vi "Knock.vi"(8 "error in (no error)":errorcluster, 11 "Node Ptr":T3 format="%.0x") -> (0 "error out":errorcluster)   [LabVIEW 2016, in "DCM System Explorer.lvlib"]
uses:
  DCM System Explorer.lvlib
  <vilib>/NI Veristand/Custom Device API/Custom Device Item Ref.ctl
  Shared/DCM Properties.vi
  Shared/DCM Constants and GUIDs.vi
  <vilib>/NI Veristand/Custom Device Tools/Custom Device Utility Library/NI VeriStand - Search for Item by Name.vi
  <vilib>/NI VeriStand/Custom Device API/Custom Device API.lvlib
  DCM Shared.lvlib
  <vilib>/NI Veristand/Custom Device Tools/Custom Device Utility Library/Custom Device Utility Library.lvlib
panel:
  in  "Settings":T1={"Knock Sensor"=[0, 0, 0, 0, 0, 0, 0, 0, 0, 0, 0, 0, 0, 0, 0, 0], "Knock Offset [CAD]"=[0.0, 0.0, 0.0, 0.0, 0.0, 0.0, 0.0, 0.0, 0.0, 0.0, 0.0, 0.0, 0.0, 0.0, 0.0, 0.0]} {"Knock Sensor" items=["Sensor 1", "Sensor 2", "Sensor 3", "Sensor 4", "Sensor 5", "Sensor 6", "Sensor 7", "Sensor 8", "Sensor 9", "Sensor 10", "Sensor 11", "Sensor 12"]}
  in  "Controls":T2={"Low Cutoff [Hz]"=5000.0, "High Cutoff [Hz]"=6000.0, "Threshold"=2.0, "Knock Start [CAD]"=0.0, "Knock End [CAD]"=0.0, "Reference End [CAD]"=0.0, "Reference Start [CAD]"=0.0} {"High Cutoff [Hz]" format="%#_6p"; "Low Cutoff [Hz]" format="%#_6p"}
  in  "Header":cluster{"Section Name":string}={"Section Name"="Knock Setup"}
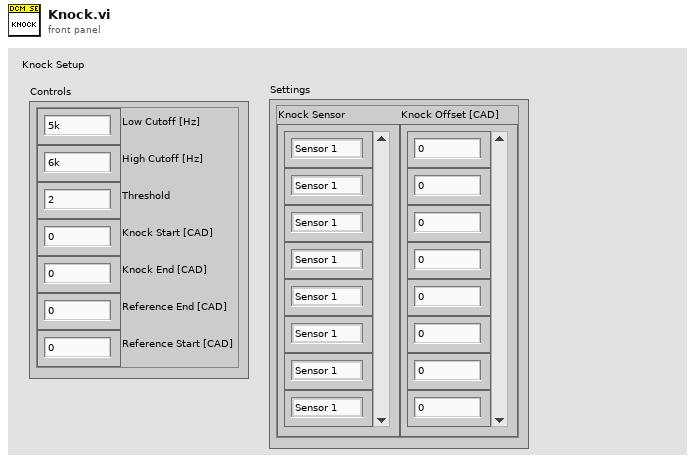
[diagram p1: front panel]
types:
  T1 = cluster{"Knock Sensor":i32[], "Knock Offset [CAD]":sgl[]}
  T2 = cluster{"Low Cutoff [Hz]":sgl, "High Cutoff [Hz]":sgl, "Threshold":sgl, "Knock Start [CAD]":sgl, "Knock End [CAD]":sgl, "Reference End [CAD]":sgl, "Reference Start [CAD]":sgl}
  T3 = typedef "Custom Device API.lvlib/Custom Device Item Ref.ctl" = u64
  T4 = typedef "DCM Shared.lvlib/Channel.ctl" = cluster{"Name":string, "Units":string, "Default":dbl, "Description":string}
  T5 = typedef "Custom Device API.lvlib/Custom Device Channel.ctl" = cluster{"Type":T6, "Units":string, "Default Value":dbl, "Faultable":bool, "Scalable":bool}
  T6 = typedef "Custom Device API.lvlib/Custom Device Channel Type.ctl" = enum16{"Input", "Output"}
  T7 = cluster{"[0]":dbl, "[1]":dbl, "[2]":dbl, "[3]":dbl, "[4]":dbl, "[5]":dbl, "[6]":dbl}
  T8 = typedef "Custom Device API.lvlib/Custom Device Commands.ctl" = enum16{"Default", "Item renamed", "Shutdown", "Dynamic button pressed"}
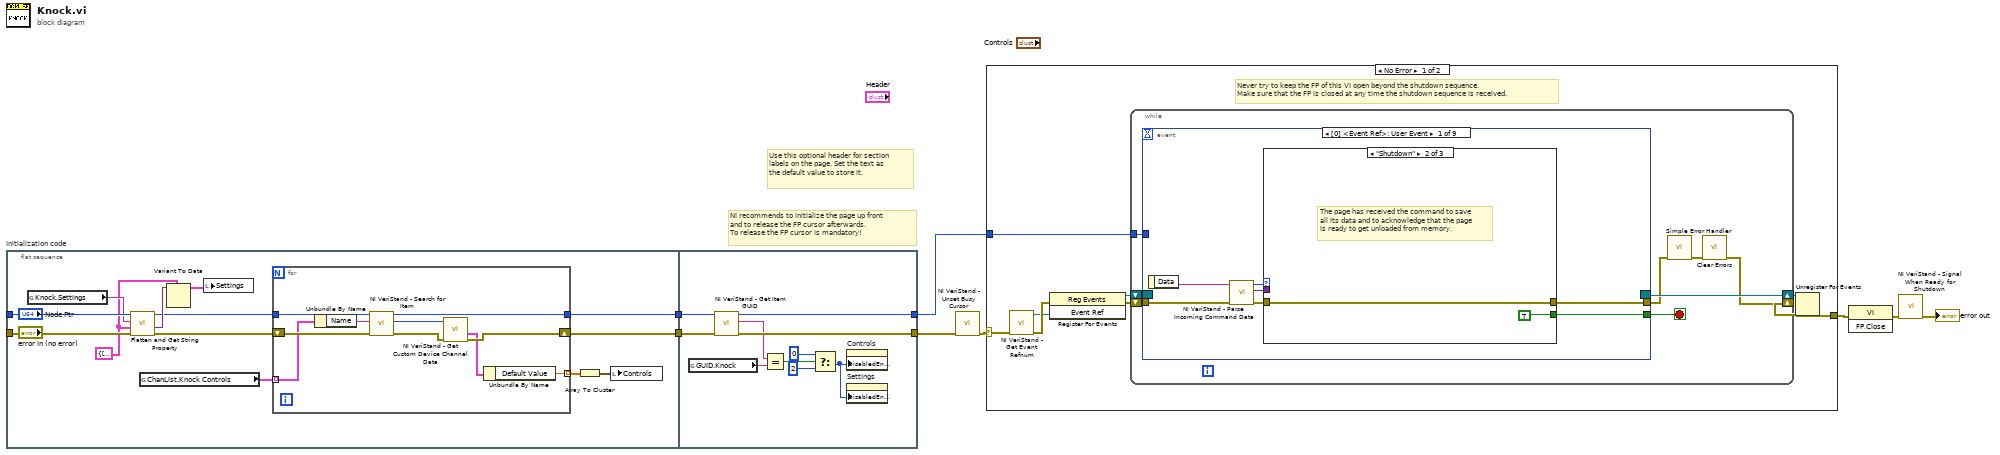
[diagram p0: block diagram]
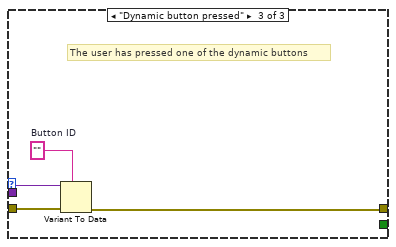
[diagram p3: hidden frame]
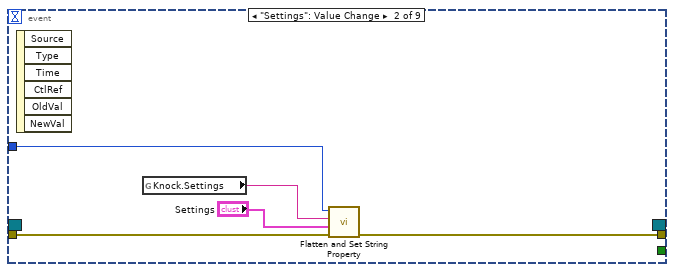
[diagram p4: hidden frame]
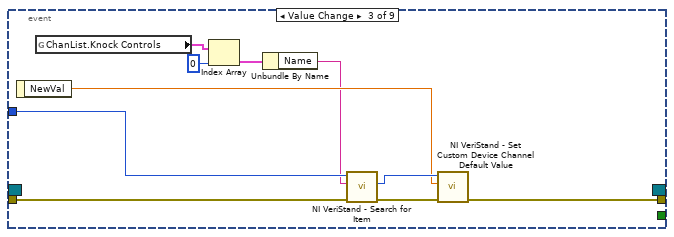
[diagram p5: hidden frame]
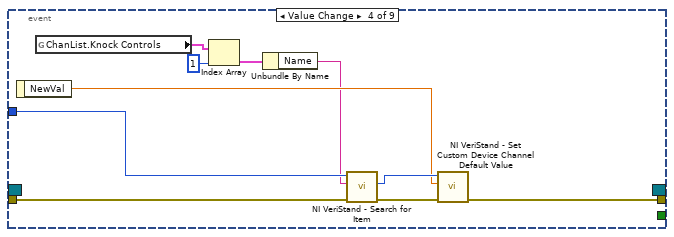
[diagram p6: hidden frame]
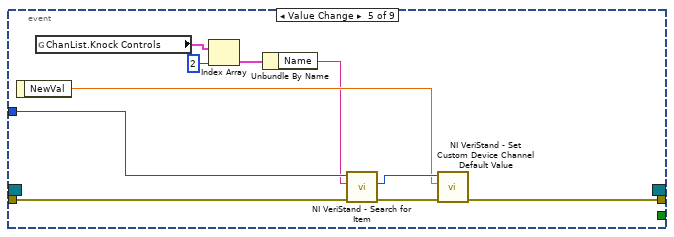
[diagram p7: hidden frame]
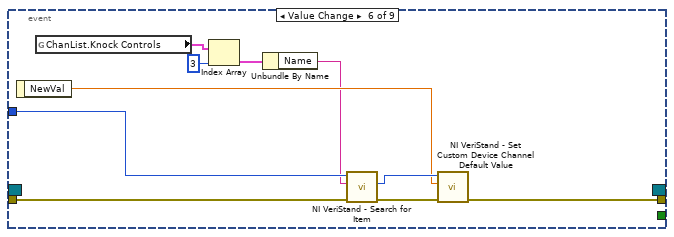
[diagram p8: hidden frame]
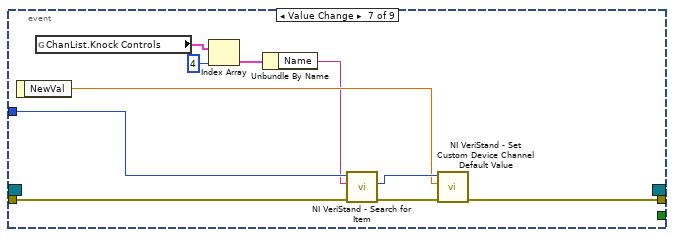
[diagram p9: hidden frame]
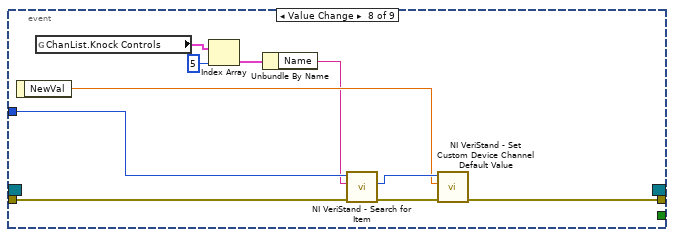
[diagram p10: hidden frame]
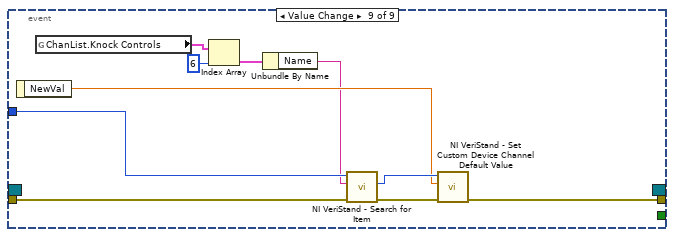
[diagram p11: hidden frame]
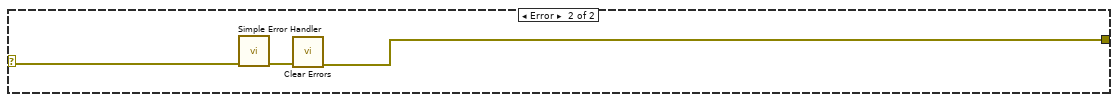
[diagram p12: hidden frame]
diagram:
  # "Use this optional header for section labels on the page. Set the text as the default value to store it."
  # "NI recommends to initialize the page up front\nand to release the FP cursor afterwards.\nTo release the FP cursor is mandatory!"
  n1 = flat-sequence "Initialization code" {
    tunnel: "error in (no error)" -> [w22]
    tunnel: "Node Ptr" -> [w21]
    tunnel: [w18] -> w2
    tunnel: [w17] -> w1
    tunnel: [w40] -> w3
    tunnel: [w41] -> w4
    tunnel: w2 -> [w43]
    tunnel: w1 -> [w42]
    frame #0 {
      w12 = T1 {"Knock Sensor"=[0, 0, 0, 0, 0, 0, 0, 0, 0, 0, 0, 0, 0, 0, 0, 0], "Knock Offset [CAD]"=[0.0, 0.0, 0.0, 0.0, 0.0, 0.0, 0.0, 0.0, 0.0, 0.0, 0.0, 0.0, 0.0, 0.0, 0.0, 0.0]} ("Settings")
      n2 = global read "DCM Properties.vi" "Knock.Settings"() -> (w20:string)
      n3 = call "Flatten and Get String Property.vi"("error in (no error)"=w22, "Default Value"=w12, "Property Name"=w20, "Section Ref in"=w21) -> ("error out"=w16:errorcluster, "Value"=w23:variant, "Section Ref out"=w19:T3)  [unwired: 5 in]
      n4 = global read "DCM Constants and GUIDs.vi" "ChanList.Knock Controls"() -> (w15:T4[])
      n5 = Variant To Data(type=w12, Variant=w23) -> (data=w11:T1)  [unwired: 1 in, 1 out]
      n6 = local write "Settings"(w11) -> ()
      n7 = for {
        tunnel: w19 -> [w33]
        tunnel: [w31] -> w18
        shift-right: [w26] -> w17
        shift-left: w16 -> [w32]
        tunnel: w15 -> [w30] mode=indexing
        tunnel: [w24] -> w14 mode=indexing
        n8 = Unbundle By Name(w30) -> ("Name"=w29:string)
        n9 = call-poly <vilib>:"NI VeriStand - Search for Item.vi"("error in"=w32, "Item Name"=w29, "Section Ref in"=w33) -> ("error out"=w28:errorcluster, "Item Ref"=w27:T3, "Section Ref out"=w31:T3)  [unwired: 5 in, 1 out]
        n10 = call <vilib>:"NI VeriStand - Get Custom Device Channel Data.vi"("error in (no error)"=w28, "Channel Ref in"=w27) -> ("error out"=w26:errorcluster, "Channel"=w25:T5)  [unwired: 4 in, 4 out]
        n11 = Unbundle By Name(w25) -> ("Default Value"=w24:dbl)
      }
      n12 = Array To Cluster(array=w14) -> (cluster=w13:T7)
      n13 = local write "Controls"(w13) -> ()
    }
    frame #1 {
      n14 = global read "DCM Constants and GUIDs.vi" "GUID.Knock"() -> (w39:string)
      n15 = call <vilib>:"NI VeriStand - Get Item GUID.vi"("error in (no error)"=w42, "Item Ref in"=w43) -> ("error out"=w40:errorcluster, "GUID"=w38:string, "Item Ref out"=w41:T3)  [unwired: 7 in]
      n16 = Equal?(x=w38, y=w39) -> (x = y?=w35:bool)
      n17 = Select(t=0, s=w35, f=2) -> (s? t:f=w34:i32)
      n18 = property on="Controls" class="Clust (strict)"("DisabledEnum"=w34) -> ()  [unwired: 2 in, 2 out]
      n19 = property on="Settings" class="Clust (strict)"("DisabledEnum"=w34) -> ()  [unwired: 2 in, 2 out]
    }
  }
  n20 = call <vilib>:"NI VeriStand - Unset Busy Cursor.vi"("error in (no error)"=w3) -> ("error out"=w6:errorcluster)  [unwired: 10 out]
  n21 = case shown="No Error" w6 {
    selector: w6 -> [w45 w152]
    tunnel: [w49 w150] -> w10
    tunnel: w4 -> [w44 _]
    frame No Error {
      # "Never try to keep the FP of this VI open beyond the shutdown sequence.\nMake sure that the FP is closed at any time the shutdown sequence is received."
      n22 = call <vilib>:"NI VeriStand - Get Event Refnum.vi"("error in (no error)"=w45) -> ("error out"=w52:errorcluster, "Event Ref"=w48:refnum<user-event>)  [unwired: 9 out]
      n23 = register-events(error in=w52, w48) -> (reference out=w46:refnum<event-registration>, error out=w47:errorcluster)  [unwired: 1 in]
      n24 = while {
        shift-right: [w54] -> w50
        shift-left: w47 -> [w59]
        shift-right: [w60] -> w51
        shift-left: w46 -> [w58]
        tunnel: w44 -> [w53]
        stop <- w57 stop-if-true
        n25 = event shown="[0] <Event Ref>: User Event" {
          selector: w58 -> [_ _ _ _ _ _ _ _ _]
          dyn-events: [_ _ _ _ _ _ _ _ _] -> w60
          timeout: _ -> [_ _ _ _ _ _ _ _ _]
          tunnel: w59 -> [w67 w79 w87 w97 w107 w117 w127 w137 w147]
          tunnel: [w63 _ _ _ _ _ _ _ _] -> w57
          tunnel: [w62 w78 w89 w99 w109 w119 w129 w139 w149] -> w56
          tunnel: w53 -> [_ w77 w88 w98 w108 w118 w128 w138 w148]
          event User Event {
            n26 = event-data() -> ("Data"=w66:string)  [unwired: 1 out]
            n27 = call <vilib>:"NI VeriStand - Parse Incoming Command Data.vi"("error in (no error)"=w67, "Incoming data"=w66) -> ("error out"=w65:errorcluster, "Outgoing data"=w61:variant, "Action"=w64:T8)  [unwired: 7 out]
            n28 = case shown="\"Shutdown\"" w64 {
              tunnel: w65 -> [w68 w69 w74]
              tunnel: [_ TRUE _] -> w63
              tunnel: [w68 w69 w71] -> w62
              tunnel: w61 -> [_ _ w73]
              frame "Default", Default {
              }
              frame "Shutdown" {
                # "The page has received the command to save all its data and to acknowledge that the page is ready to get unloaded from memory."
              }
              frame "Dynamic button pressed" {
                w72 = ""  # Button ID
                # "The user has pressed one of the dynamic buttons"
                n29 = Variant To Data(error in=w74, type=w72, Variant=w73) -> (error out=w71:errorcluster)  [unwired: 1 out]
              }
            }
          }
          event "Settings": Value Change {
            n30 = event-data() -> ()  [unwired: 7 out]
            n31 = global read "DCM Properties.vi" "Knock.Settings"() -> (w76:string)
            n32 = call "Flatten and Set String Property.vi"("error in (no error)"=w79, "Value"="Settings", "Property Name"=w76, "Section Ref in"=w77) -> ("error out"=w78:errorcluster)  [unwired: 6 in, 1 out]
          }
          event "Controls.Low Cutoff [Hz]": Value Change {
            n33 = event-data() -> ("NewVal"=w84:sgl)  [unwired: 1 out]
            n34 = global read "DCM Constants and GUIDs.vi" "ChanList.Knock Controls"() -> (w83:T4[])
            n35 = Index Array(array=w83, index=0) -> (element=w81:T4)
            n36 = Unbundle By Name(w81) -> ("Name"=w80:string)
            n37 = call-poly <vilib>:"NI VeriStand - Search for Item.vi"("error in"=w87, "Item Name"=w80, "Section Ref in"=w88) -> ("error out"=w86:errorcluster, "Item Ref"=w85:T3)  [unwired: 5 in, 2 out]
            n38 = call <vilib>:"NI VeriStand - Set Custom Device Channel Default Value.vi"("error in (no error)"=w86, "Default Value"=w84, "Channel Ref in"=w85) -> ("error out"=w89:errorcluster)  [unwired: 7 in, 1 out]
          }
          event "Controls.High Cutoff [Hz]": Value Change {
            n39 = event-data() -> ("NewVal"=w94:sgl)  [unwired: 1 out]
            n40 = global read "DCM Constants and GUIDs.vi" "ChanList.Knock Controls"() -> (w93:T4[])
            n41 = Index Array(array=w93, index=1) -> (element=w91:T4)
            n42 = Unbundle By Name(w91) -> ("Name"=w90:string)
            n43 = call-poly <vilib>:"NI VeriStand - Search for Item.vi"("error in"=w97, "Item Name"=w90, "Section Ref in"=w98) -> ("error out"=w96:errorcluster, "Item Ref"=w95:T3)  [unwired: 5 in, 2 out]
            n44 = call <vilib>:"NI VeriStand - Set Custom Device Channel Default Value.vi"("error in (no error)"=w96, "Default Value"=w94, "Channel Ref in"=w95) -> ("error out"=w99:errorcluster)  [unwired: 7 in, 1 out]
          }
          event "Controls.Threshold": Value Change {
            n45 = event-data() -> ("NewVal"=w104:sgl)  [unwired: 1 out]
            n46 = global read "DCM Constants and GUIDs.vi" "ChanList.Knock Controls"() -> (w103:T4[])
            n47 = Index Array(array=w103, index=2) -> (element=w101:T4)
            n48 = Unbundle By Name(w101) -> ("Name"=w100:string)
            n49 = call-poly <vilib>:"NI VeriStand - Search for Item.vi"("error in"=w107, "Item Name"=w100, "Section Ref in"=w108) -> ("error out"=w106:errorcluster, "Item Ref"=w105:T3)  [unwired: 5 in, 2 out]
            n50 = call <vilib>:"NI VeriStand - Set Custom Device Channel Default Value.vi"("error in (no error)"=w106, "Default Value"=w104, "Channel Ref in"=w105) -> ("error out"=w109:errorcluster)  [unwired: 7 in, 1 out]
          }
          event "Controls.Knock Start [CAD]": Value Change {
            n51 = event-data() -> ("NewVal"=w114:sgl)  [unwired: 1 out]
            n52 = global read "DCM Constants and GUIDs.vi" "ChanList.Knock Controls"() -> (w113:T4[])
            n53 = Index Array(array=w113, index=3) -> (element=w111:T4)
            n54 = Unbundle By Name(w111) -> ("Name"=w110:string)
            n55 = call-poly <vilib>:"NI VeriStand - Search for Item.vi"("error in"=w117, "Item Name"=w110, "Section Ref in"=w118) -> ("error out"=w116:errorcluster, "Item Ref"=w115:T3)  [unwired: 5 in, 2 out]
            n56 = call <vilib>:"NI VeriStand - Set Custom Device Channel Default Value.vi"("error in (no error)"=w116, "Default Value"=w114, "Channel Ref in"=w115) -> ("error out"=w119:errorcluster)  [unwired: 7 in, 1 out]
          }
          event "Controls.Knock End [CAD]": Value Change {
            n57 = event-data() -> ("NewVal"=w124:sgl)  [unwired: 1 out]
            n58 = global read "DCM Constants and GUIDs.vi" "ChanList.Knock Controls"() -> (w123:T4[])
            n59 = Index Array(array=w123, index=4) -> (element=w121:T4)
            n60 = Unbundle By Name(w121) -> ("Name"=w120:string)
            n61 = call-poly <vilib>:"NI VeriStand - Search for Item.vi"("error in"=w127, "Item Name"=w120, "Section Ref in"=w128) -> ("error out"=w126:errorcluster, "Item Ref"=w125:T3)  [unwired: 5 in, 2 out]
            n62 = call <vilib>:"NI VeriStand - Set Custom Device Channel Default Value.vi"("error in (no error)"=w126, "Default Value"=w124, "Channel Ref in"=w125) -> ("error out"=w129:errorcluster)  [unwired: 7 in, 1 out]
          }
          event "Controls.Reference Start [CAD]": Value Change {
            n63 = event-data() -> ("NewVal"=w134:sgl)  [unwired: 1 out]
            n64 = global read "DCM Constants and GUIDs.vi" "ChanList.Knock Controls"() -> (w133:T4[])
            n65 = Index Array(array=w133, index=5) -> (element=w131:T4)
            n66 = Unbundle By Name(w131) -> ("Name"=w130:string)
            n67 = call-poly <vilib>:"NI VeriStand - Search for Item.vi"("error in"=w137, "Item Name"=w130, "Section Ref in"=w138) -> ("error out"=w136:errorcluster, "Item Ref"=w135:T3)  [unwired: 5 in, 2 out]
            n68 = call <vilib>:"NI VeriStand - Set Custom Device Channel Default Value.vi"("error in (no error)"=w136, "Default Value"=w134, "Channel Ref in"=w135) -> ("error out"=w139:errorcluster)  [unwired: 7 in, 1 out]
          }
          event "Controls.Reference End [CAD]": Value Change {
            n69 = event-data() -> ("NewVal"=w144:sgl)  [unwired: 1 out]
            n70 = global read "DCM Constants and GUIDs.vi" "ChanList.Knock Controls"() -> (w143:T4[])
            n71 = Index Array(array=w143, index=6) -> (element=w141:T4)
            n72 = Unbundle By Name(w141) -> ("Name"=w140:string)
            n73 = call-poly <vilib>:"NI VeriStand - Search for Item.vi"("error in"=w147, "Item Name"=w140, "Section Ref in"=w148) -> ("error out"=w146:errorcluster, "Item Ref"=w145:T3)  [unwired: 5 in, 2 out]
            n74 = call <vilib>:"NI VeriStand - Set Custom Device Channel Default Value.vi"("error in (no error)"=w146, "Default Value"=w144, "Channel Ref in"=w145) -> ("error out"=w149:errorcluster)  [unwired: 7 in, 1 out]
          }
        }
        n75 = call <vilib>:"Simple Error Handler.vi"("error in (no error)"=w56) -> ("error out"=w55:errorcluster)  [unwired: 1 in, 7 out]
        n76 = call <vilib>:"Clear Errors.vi"("error in (no error)"=w55) -> ("error out"=w54:errorcluster)  [unwired: 1 in, 5 out]
      }
      n77 = Unregister For Events(event registration refnum=w51, error in=w50) -> (error out=w49:errorcluster)
    }
    frame Error {
      n78 = call <vilib>:"Simple Error Handler.vi"("error in (no error)"=w152) -> ("error out"=w151:errorcluster)  [unwired: 1 in, 7 out]
      n79 = call <vilib>:"Clear Errors.vi"("error in (no error)"=w151) -> ("error out"=w150:errorcluster)  [unwired: 1 in, 5 out]
    }
  }
  n80 = invoke class="VI" method="FP.Close"(error in=w10) -> (error out=w9:errorcluster)  [unwired: 2 in, 2 out]
  n81 = call <vilib>:"NI VeriStand - Signal When Ready for Shutdown.vi"("error in (no error)"=w9) -> ("error out"=→"error out":errorcluster)  [unwired: 10 out]
